vi "Publish Data.vi"(6 "Publish Time (Use Current Time)":timestamp, 8 "error in (no error)":errorcluster, 9 "Data to Publish":variant, 10 "Datum Name":string, 11 "IViewModel In":refnum<class "IViewModel.lvclass">) -> (0 "error out":errorcluster, 3 "IViewModel Out":refnum<class "IViewModel.lvclass">)   [LabVIEW 2020, in "MVA Framework.lvlib" / "IViewModel.lvlib" / "IViewModel.lvclass"]
doc: "发布数据"
uses:
  IViewModel.lvclass
  mva-core/Source/IObserver/IObserver/IObserver.lvclass/IObserver.ctl
  IViewModel.lvclass/IViewModel.ctl
  mva-core/Source/IMediator/PublishRequest/PublishRequest.lvclass
  mva-core/Source/IMediator/PublishRequest/PublishRequest.lvclass/PublishRequest.ctl
  mva-core/Source/IMediator/IMediator Messages/Publish Msg/Publish Msg.lvclass/Publish Msg.ctl
  composed-af-messages/Source/RoundTripMessage/RoundTripMessage.lvclass/RoundTripMessage.ctl
  <vilib>/ActorFramework/Message Enqueuer/Message Enqueuer.lvclass/Message Enqueuer.ctl
  composed-af-messages/Source/RoundTripMessage/Return Round-Trip Message.vi
  <vilib>/ActorFramework/Message Enqueuer/Enqueue.vi
  mva-core/Source/IMediator/IMediator Messages/Publish Msg/Publish Msg.lvclass
  composed-af-messages/Source/RoundTripMessage/RoundTripMessage.lvclass
  C:/Program Files/National Instruments/LabVIEW 2020/vi.lib/ActorFramework/Message/Message.lvclass
  <vilib>/Utility/error.llb/Error Cluster From Error Code.vi
  <vilib>/ActorFramework/Message Priority Queue/Priority Enqueue.vi
  mva-core/Source/IObserver/IObserver/IObserver.lvclass
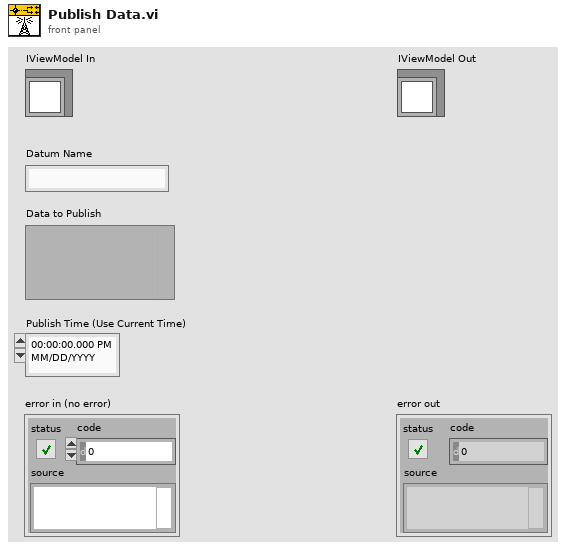
[diagram p1: front panel]
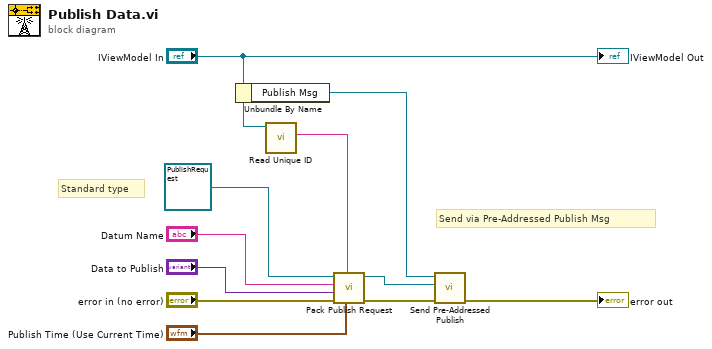
[diagram p0: block diagram]
diagram:
  # "Standard type"
  # "Send via Pre-Addressed Publish Msg"
  n1 = Unbundle By Name("IViewModel In") -> ("Publish Msg"=w11:refnum<class "Publish Msg.lvclass">)
  n2 = call "Read Unique ID.vi"("IObserver In"="IViewModel In") -> ("Unique ID"=w7:string)  [unwired: 10 in]
  n3 = call "Pack Publish Request.vi"("Publication Time (Use Current Time)"="Publish Time (Use Current Time)", "Publisher ID"=w7, "error in (no error)"="error in (no error)", "Value"="Data to Publish", "Datum Name"="Datum Name", "PublishRequest In"=refnum<class "PublishRequest.lvclass"> refnum) -> ("error out"=w5:errorcluster, "PublishRequest Out"=w8:refnum<class "PublishRequest.lvclass">)  [unwired: 4 in]
  n4 = call "Send Pre-Addressed Publish.vi"("error in (no error)"=w5, "PublishRequest"=w8, "Publish Message"=w11) -> ("error out"=→"error out":errorcluster)  [unwired: 8 in]
  "IViewModel Out" <- "IViewModel In"
